vi "Transmit Transfer Data.vi"(5 "transfer id":i32, 7 "transfer group id":i32, 8 "error in":errorcluster, 9 "transfer data":u8[](array[numeric]), 11 "RDMA Transceiver in":refnum<class "RDMA Transceiver.lvclass">) -> (0 "error out":errorcluster, 1 "timed out?":bool, 3 "RDMA Transceiver out":refnum<class "RDMA Transceiver.lvclass">)   [LabVIEW 2020, in "RDMA.lvlib" / "RDMA Transceiver.lvclass"]
doc: "Writes transfer data to RDMA buffer"
uses:
  RDMA Transceiver.lvclass
  RDMA Transceiver.lvclass/RDMA Transceiver.ctl
  <vilib>/Utility/error.llb/Clear Errors.vi
  <vilib>/rdma/rdma.llb/RDMA Acquire Send Buffer.vi
  <vilib>/rdma/rdma.llb/RDMA Acquire Send Buffer U8.vi
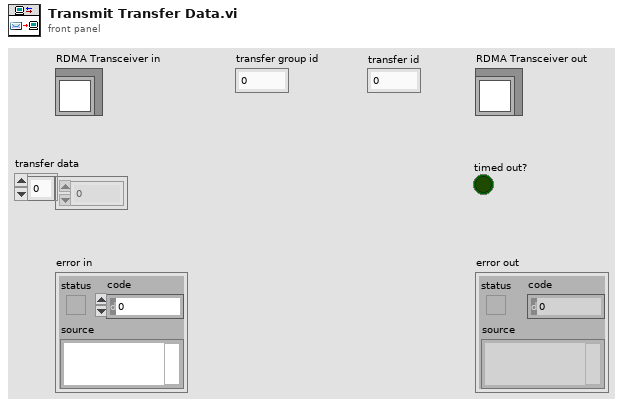
[diagram p1: front panel]
types:
  T1 = typedef "RDMA.lvlib/RDMA Transceiver.lvclass/Transfer Group Parameters.ctl" = cluster{"transfers":T2[]}
  T2 = typedef "RDMA.lvlib/RDMA Transceiver.lvclass/Transfer Parameters.ctl" = cluster{"connected session":refnum<k21>, "listener session":refnum<k21>}
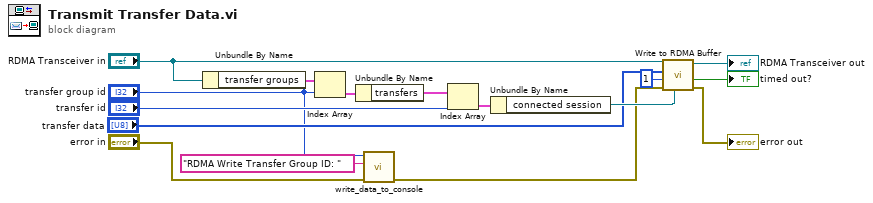
[diagram p0: block diagram]
diagram:
  n1 = Unbundle By Name("RDMA Transceiver in") -> ("transfer groups"=w16:T1[])
  n2 = Index Array(array=w16, index="transfer group id") -> (element=w15:T1)
  n3 = Unbundle By Name(w15) -> ("transfers"=w13:T2[])
  n4 = call "write_data_to_console.vi"("error in"="error in", "Tag"="RDMA Write Transfer Group ID: ", "Data"="transfer group id") -> ("error out"=w3:errorcluster)  [unwired: 8 in]
  n5 = Index Array(array=w13, index="transfer id") -> (element=w14:T2)
  n6 = Unbundle By Name(w14) -> ("connected session"=w6:refnum<k21>)
  n7 = call "Write to RDMA Buffer.vi"("rdma session"=w6, "error in"=w3, "timeout ms (25000)"=1, "data"="transfer data", "RDMA Transceiver in"="RDMA Transceiver in") -> ("error out"=→"error out":errorcluster, "timed out?"=→"timed out?":bool, "RDMA Transceiver out"=→"RDMA Transceiver out":refnum<class "RDMA Transceiver.lvclass">)  [unwired: 4 in]
